vi "FA_SortConfigData.vi"(11 "Config In":T1) -> (3 "Config":T1)   [LabVIEW 2014, in "FA_NativeTypes.lvlib"]
doc: "Sorts the parameter name/value pairs based on a prepended number and removes this number"
uses:
  FA_NativeTypes.lvlib
  FA_Config.ctl
  FA_LocalStore API/source/VI Source/FA_LSSpecialTypes.ctl
  FA_LocalStore API/source/VI Source/FA_LocalStore.lvlib
panel:
  out "Error Out":errorcluster
  in  "Error In":errorcluster
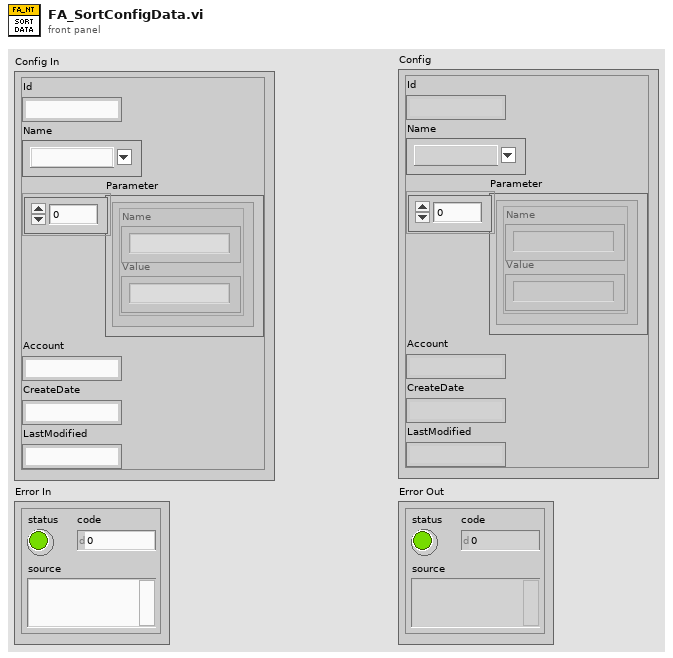
[diagram p1: front panel]
types:
  T1 = typedef "FA_NativeTypes.lvlib/FA_Config.ctl" = cluster{"Id":string, "Name":T2, "Parameter":cluster{"Name":string, "Value":string}[], "Account":string, "CreateDate":string, "LastModified":string}
  T2 = typedef "FA_LocalStore.lvlib/FA_LSSpecialTypes.ctl" = string
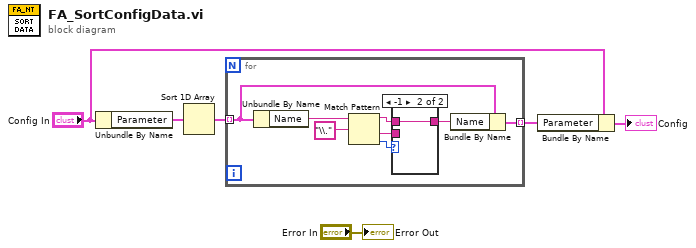
[diagram p0: block diagram]
diagram:
  n1 = Unbundle By Name("Config In") -> ("Parameter"=w6:cluster{"Name":string, "Value":string}[])
  n2 = Sort 1D Array(array=w6) -> (sorted array=w2:cluster{"Name":string, "Value":string}[])
  n3 = for {
    tunnel: w2 -> [w14] mode=indexing
    tunnel: [w13] -> w1 mode=indexing
    n4 = Unbundle By Name(w14) -> ("Name"=w12:string)
    n5 = Match Pattern(string=w12, regular expression="\\.") -> (before substring=w9:string, after substring=w8:string, offset past match=w10:i32)  [unwired: 1 in, 1 out]
    n6 = case shown="-1" w10 {
      tunnel: w9 -> [_ w16]
      tunnel: w8 -> [w15 _]
      tunnel: [w15 w16] -> w7
      frame 0, Default {
      }
      frame -1 {
      }
    }
    n7 = Bundle By Name(cluster=w14, "Name"=w7) -> (w13:cluster{"Name":string, "Value":string})
  }
  n8 = Bundle By Name(cluster="Config In", "Parameter"=w1) -> (→"Config":T1)
  "Error Out" <- "Error In"
